vi "Query Chan Parameters (Input).vi"(7 "Channel (1: Chan A)":i32(ring)=1 items=["Channel A"=1, "Channel B"=2, "Channel C"=3, "Channel D"=4, "Channel E"=5, "Channel F"=6, "Channel G"=7, "Channel H"=8], 8 "error in (no error)":errorcluster, 11 "VISA resource name":refnum<visa-resource-name>) -> (0 "error out":errorcluster, 2 "Input Parameters":T1 {"Sync Source" items=["System (To)", "Channel A", "Channel B", "Channel C", "Channel D", "Channel E", "Channel F", "Channel G", "Channel H"]}, 3 "VISA resource name out":refnum<visa-resource-name>)   [LabVIEW 2019, in "Quantum Composers 9000 Series.lvlib"]
doc: "This VI is used to read the input configuration of the selected channel."
uses:
  Quantum Composers 9000 Series.lvlib
panel:
  # "The \"Gate Mode\" is currently only utilized by 9520/9530 instruments.  When controlling a 9520/9530,  the \"Gate Logic\" disabled setting is ignored."
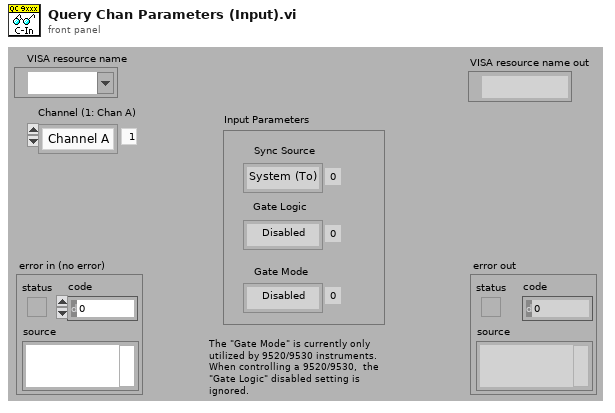
[diagram p1: front panel]
types:
  T1 = cluster{"Gate Logic":enum16{"Disabled", "Low", "High"}, "Sync Source":i32, "Gate Mode":enum16{"Disabled", "Pulse Inhibit", "Output Inhibit"}}
  T2 = enum16{"Disabled", "Pulse Inhibit", "Output Inhibit"}
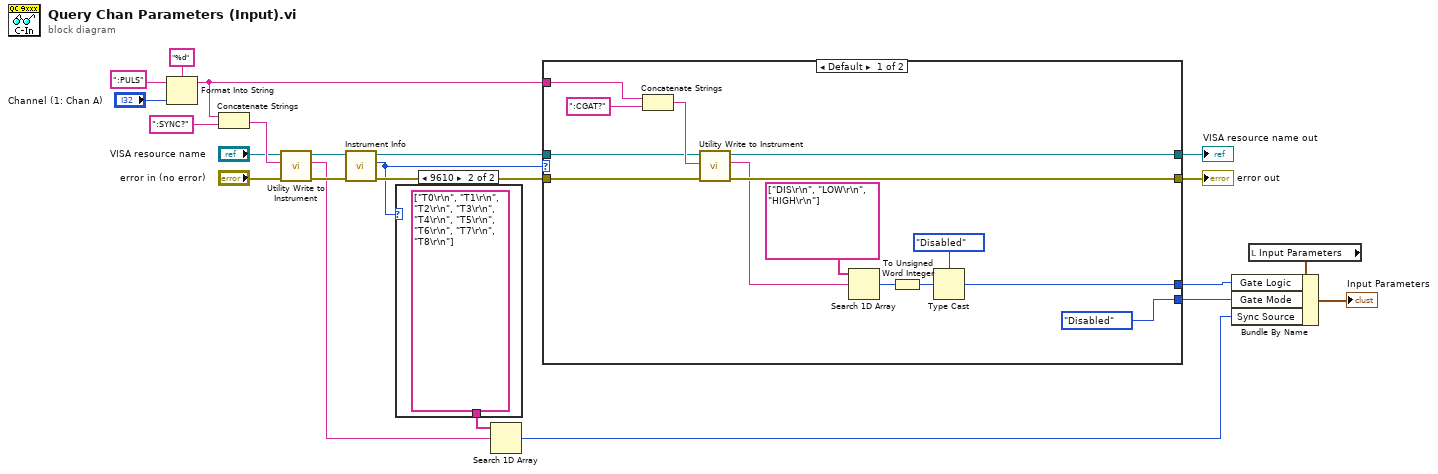
[diagram p0: block diagram]
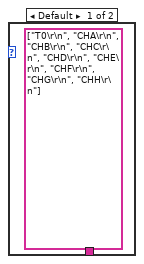
[diagram p2: hidden frame]
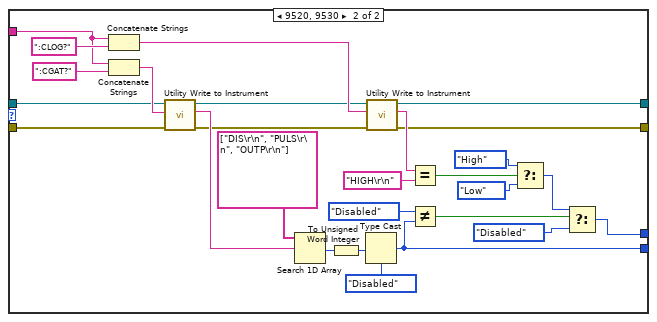
[diagram p3: hidden frame]
diagram:
  n1 = Format Into String(format string="%d", initial string=":PULS", "Channel (1: Chan A)") -> (resulting string=w5:string)  [unwired: 1 in, 1 out]
  n2 = Concatenate Strings(w5, ":SYNC?") -> (w10:string)
  n3 = call "Utility Write to Instrument.vi"("error in (no error)"="error in (no error)", "Write Buffer"=w10, "VISA resource name"="VISA resource name") -> ("error out"=w8:errorcluster, "Read Buffer"=w6:string, "VISA resource name out"=w7:refnum<visa-resource-name>)  [unwired: 6 in]
  n4 = call "Instrument Info.vi"("error in (no error)"=w8, "VISA resource name"=w7) -> ("error out"=w14:errorcluster, "Instr Model"=w1:u32, "VISA resource name out"=w13:refnum<visa-resource-name>)  [unwired: 6 in, 1 out]
  n5 = case shown="9610" w1 {
    tunnel: [string[] ["T0\r\n", "CHA\r\n", "CHB\r\n", "CHC\r\n", "CHD\r\n", "CHE\r\n", "CHF\r\n", "CHG\r\n", "CHH\r\n"] string[] ["T0\r\n", "T1\r\n", "T2\r\n", "T3\r\n", "T4\r\n", "T5\r\n", "T6\r\n", "T7\r\n", "T8\r\n"]] -> w11
    frame Default {
    }
    frame 9610 {
    }
  }
  n6 = Search 1D Array(1D array=w11, element=w6) -> (index of element=w2:i32)  [unwired: 1 in]
  n7 = case shown="Default" w1 {
    tunnel: w5 -> [w37 w60]
    tunnel: w13 -> [w28 w56]
    tunnel: w14 -> [w29 w57]
    tunnel: [w35 w50] -> w19
    tunnel: [w34 w51] -> w18
    tunnel: [w31 w41] -> w15
    tunnel: [T2."Disabled" ("Gate Mode") w48] -> w12
    frame Default {
      n8 = Concatenate Strings(w37, ":CGAT?") -> (w36:string)
      n9 = call "Utility Write to Instrument.vi"("error in (no error)"=w29, "Write Buffer"=w36, "VISA resource name"=w28) -> ("error out"=w34:errorcluster, "Read Buffer"=w32:string, "VISA resource name out"=w35:refnum<visa-resource-name>)  [unwired: 6 in]
      n10 = Search 1D Array(1D array=string[] ["DIS\r\n", "LOW\r\n", "HIGH\r\n"], element=w32) -> (index of element=w26:i32)  [unwired: 1 in]
      n11 = To Unsigned Word Integer(number=w26) -> (unsigned 16bit integer=w25:u16)
      n12 = Type Cast(type=enum16{"Disabled", "Low", "High"}."Disabled" ("Gate Logic"), x=w25) -> (*(type *) &x=w31:enum16{"Disabled", "Low", "High"})
    }
    frame 9520, 9530 {
      n13 = Concatenate Strings(w60, ":CLOG?") -> (w59:string)
      n14 = Concatenate Strings(w60, ":CGAT?") -> (w64:string)
      n15 = call "Utility Write to Instrument.vi"("error in (no error)"=w57, "Write Buffer"=w64, "VISA resource name"=w56) -> ("error out"=w55:errorcluster, "Read Buffer"=w62:string, "VISA resource name out"=w54:refnum<visa-resource-name>)  [unwired: 6 in]
      n16 = Search 1D Array(1D array=string[] ["DIS\r\n", "PULS\r\n", "OUTP\r\n"], element=w62) -> (index of element=w39:i32)  [unwired: 1 in]
      n17 = To Unsigned Word Integer(number=w39) -> (unsigned 16bit integer=w40:u16)
      n18 = Type Cast(type=T2."Disabled" ("Gate Mode"), x=w40) -> (*(type *) &x=w48:T2)
      n19 = call "Utility Write to Instrument.vi"("error in (no error)"=w55, "Write Buffer"=w59, "VISA resource name"=w54) -> ("error out"=w51:errorcluster, "Read Buffer"=w53:string, "VISA resource name out"=w50:refnum<visa-resource-name>)  [unwired: 6 in]
      n20 = Equal?(x=w53, y="HIGH\r\n") -> (x = y?=w47:bool)
      n21 = Not Equal?(x=T2."Disabled" ("Gate Mode"), y=w48) -> (x != y?=w46:bool)
      n22 = Select(t=enum16{"Disabled", "Low", "High"}."High" ("Gate Logic"), s=w47, f=enum16{"Disabled", "Low", "High"}."Low" ("Gate Logic")) -> (s? t:f=w44:enum16{"Disabled", "Low", "High"})
      n23 = Select(t=w44, s=w46, f=enum16{"Disabled", "Low", "High"}."Disabled" ("Gate Logic")) -> (s? t:f=w41:enum16{"Disabled", "Low", "High"})
    }
  }
  "VISA resource name out" <- w19
  "error out" <- w18
  n24 = local read "Input Parameters"() -> (w16:T1)
  n25 = Bundle By Name(cluster=w16, "Gate Logic"=w15, "Gate Mode"=w12, "Sync Source"=w2) -> (→"Input Parameters":T1)
